vi "Main Coefficiente binomiale.vi"() -> ()   [LabVIEW 2021]
panel:
  out "Coefficiente binomiale":dbl
  in  "k":u8=1 min=1 step=1
  in  "n":u8=1 min=1 step=1
  # "n!\nCoefficiente binomiale=------------------\n                                              k! (n-k)!"
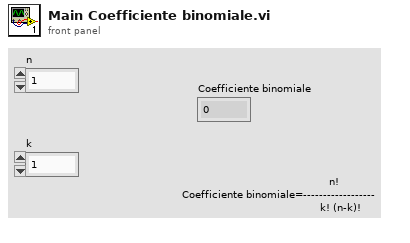
[diagram p1: front panel]
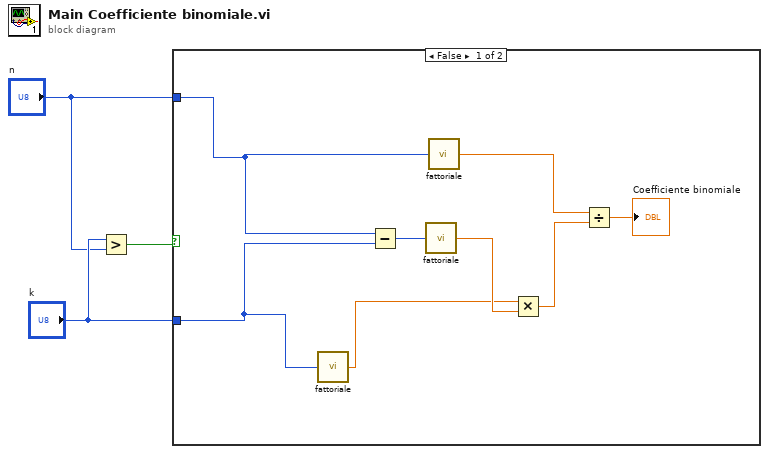
[diagram p0: block diagram]
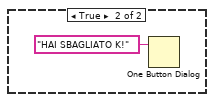
[diagram p2: hidden frame]
diagram:
  n1 = Greater?(x="k", y="n") -> (0:w1:bool)
  n2 = case shown="False" w1 {
    tunnel: "k" -> [w6 _]
    tunnel: "n" -> [w5 _]
    frame False {
      n3 = call "fattoriale.vi"("n"=w6) -> ("n!"=w9:dbl)
      n4 = Subtract(x=w5, y=w6) -> (x-y=w11:u8)
      n5 = call "fattoriale.vi"("n"=w11) -> ("n!"=w10:dbl)
      n6 = call "fattoriale.vi"("n"=w5) -> ("n!"=w8:dbl)
      n7 = Multiply(x=w9, y=w10) -> (x*y=w7:dbl)
      n8 = Divide(x=w8, y=w7) -> (x/y=→"Coefficiente binomiale":dbl)
    }
    frame True {
      n9 = One Button Dialog(message="HAI SBAGLIATO K!") -> ()  [unwired: 1 in, 1 out]
    }
  }
